vi "Write myNum.vi"(8 "error in (no error)":errorcluster, 10 "myNum":dbl, 11 "Test3 in":refnum<class "Class3.lvclass">) -> (0 "error out":errorcluster, 3 "Test3 out":refnum<class "Class3.lvclass">)   [LabVIEW 2020, in "Class3.lvclass"]
doc: "GCraftsman JSON Object Serialization Toolkit\nwww.GCraftsman.com\nCopyright (c) 2017, GCraftsman"
uses:
  Class3.lvclass
  Class3.lvclass/Class3.ctl
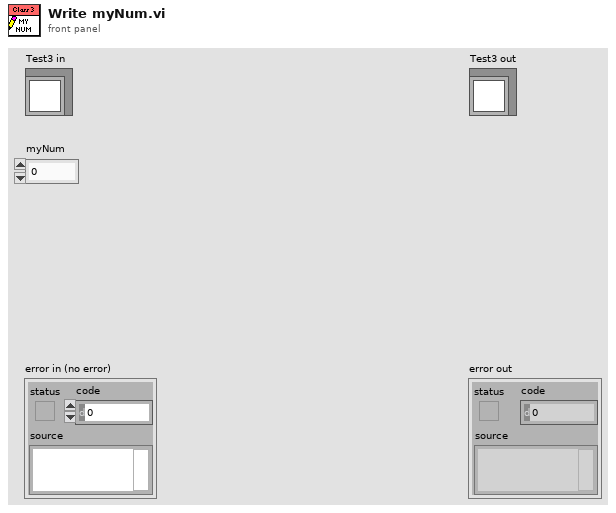
[diagram p1: front panel]
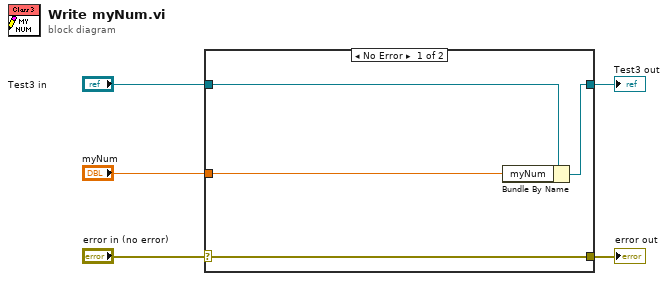
[diagram p0: block diagram]
diagram:
  n1 = case shown="No Error" "error in (no error)" {
    selector: "error in (no error)" -> [w9 w10]
    tunnel: [w9 w10] -> w4
    tunnel: [w7 w11] -> w2
    tunnel: "Test3 in" -> [w8 w11]
    tunnel: "myNum" -> [w6 _]
    frame No Error {
      n2 = Bundle By Name(cluster=w8, "myNum"=w6) -> (w7:refnum<class "Class3.lvclass">)
    }
    frame Error {
    }
  }
  "error out" <- w4
  "Test3 out" <- w2
